vi "lectura acelerometro.vi"(4 "read buffer":string) -> (0 "Acelerómetro Z":sgl[](array[numeric]), 1 "Acelerómetro Y":sgl[](array[numeric]), 2 "Acelerómetro X":sgl[](array[numeric]))   [LabVIEW 2020]
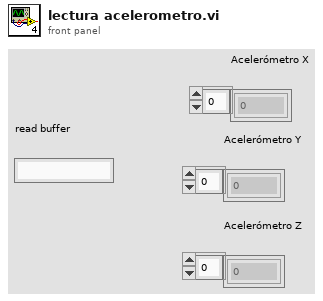
[diagram p1: front panel]
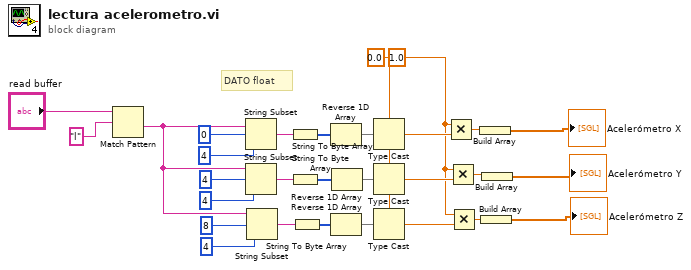
[diagram p0: block diagram]
diagram:
  w7 = 1.0
  w12 = sgl 0.0
  # "DATO float"
  n1 = Match Pattern(string="read buffer", regular expression="l") -> (after substring=w4:string)  [unwired: 1 in, 3 out]
  n2 = String Subset(string=w4, offset (0)=0, length (rest)=4 ("length (rest)")) -> (substring=w21:string)
  n3 = String Subset(string=w4, offset (0)=4, length (rest)=4 ("length (rest)")) -> (substring=w20:string)
  n4 = String Subset(string=w4, offset (0)=8, length (rest)=4 ("length (rest)")) -> (substring=w19:string)
  n5 = String To Byte Array(string=w21) -> (unsigned byte array=w18:u8[])
  n6 = String To Byte Array(string=w20) -> (unsigned byte array=w14:u8[])
  n7 = String To Byte Array(string=w19) -> (unsigned byte array=w13:u8[])
  n8 = Reverse 1D Array(array=w18) -> (reversed array=w17:u8[])
  n9 = Reverse 1D Array(array=w13) -> (reversed array=w15:u8[])
  n10 = Reverse 1D Array(array=w14) -> (reversed array=w16:u8[])
  n11 = Type Cast(type=w12, x=w17) -> (*(type *) &x=w10:sgl)
  n12 = Type Cast(type=w12, x=w16) -> (*(type *) &x=w9:sgl)
  n13 = Type Cast(type=w12, x=w15) -> (*(type *) &x=w8:sgl)
  n14 = Multiply(x=w7, y=w10) -> (x*y=w11:dbl)
  n15 = Multiply(x=w7, y=w9) -> (x*y=w6:dbl)
  n16 = Multiply(x=w7, y=w8) -> (x*y=w5:dbl)
  n17 = Build Array(w11) -> (→"Acelerómetro X":dbl[])
  n18 = Build Array(w5) -> (→"Acelerómetro Z":dbl[])
  n19 = Build Array(w6) -> (→"Acelerómetro Y":dbl[])
